vi "Read VI name.vi"(8 "error in":errorcluster, 11 "UI Reference configuration in":refnum<class "UI Reference configuration.lvclass">) -> (0 "error out":errorcluster, 2 "VI name":string, 3 "UI Reference configuration out":refnum<class "UI Reference configuration.lvclass">)   [LabVIEW 2013, in "UI Reference configuration.lvclass"]
uses:
  UI Reference configuration.lvclass
  UI Reference configuration.lvclass/UI Reference configuration.ctl
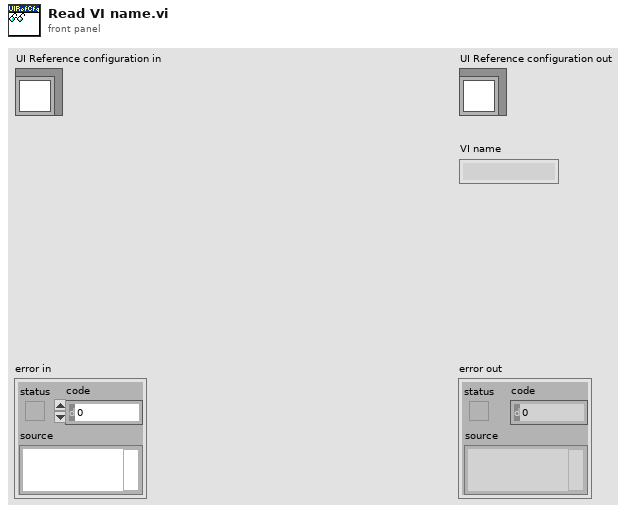
[diagram p1: front panel]
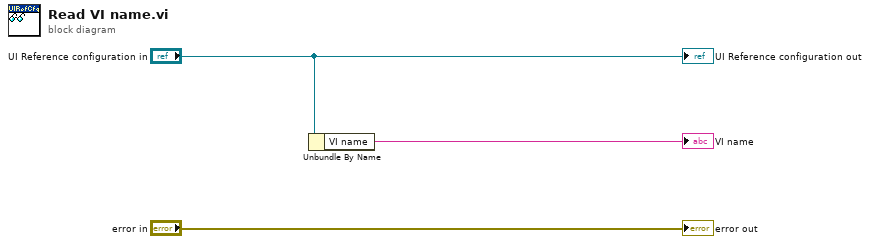
[diagram p0: block diagram]
diagram:
  n1 = Unbundle By Name("UI Reference configuration in") -> ("VI name"=→"VI name":string)
  "error out" <- "error in"
  "UI Reference configuration out" <- "UI Reference configuration in"
